vi "TDF - Time Varying Filter - Gabor.vi"(0 "reference in":refnum<class "GSwFormDSP.lvclass">, 5 "error in (no error)":errorcluster, 6 "Anotate Signal Name":bool=TRUE) -> (14 "reference in":refnum<class "GSwFormDSP.lvclass">, 19 "error out":errorcluster)   [LabVIEW 2022 SP3, in "GSwFormDSP.lvclass"]
uses:
  GSwFormDSP.lvclass
  <vilib>/addons/Time Frequency Analysis/Application.llb/TFA Time Varying Filter (Waveform).vi
  <vilib>/addons/_Advanced Signal Processing/NI_AdvSigProcTFA.lvlib
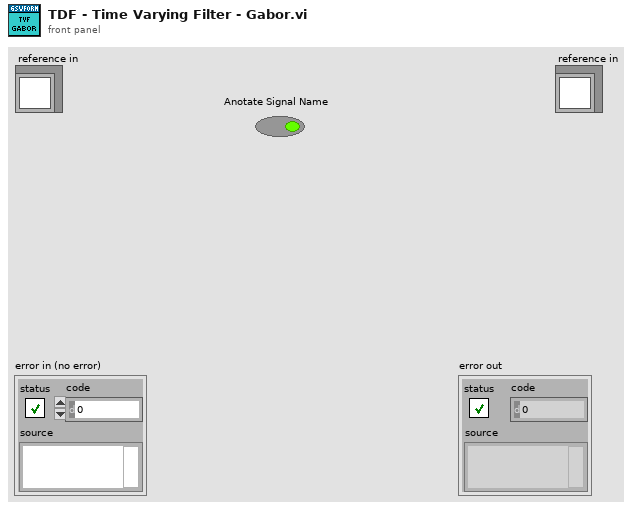
[diagram p1: front panel]
types:
  T1 = typedef "GSwFormDSP.lvclass/ObjectAttributes.ctl" = cluster{"Wform Ref":refnum<data-value>, "Nb Signals":i32, "Spectral Function Parameters":T2, "FFT":waveform(cdb)[], "Nb FFT":i32, "Nb Averages":i32[], "Reference Indexes":i32[], "Response Indexes":i32[], "Coherence":waveform(dbl)[], "TDF Parameters":T4, "DAQ":cluster{"Duration (sec)":dbl, "Buffer Size (Samples)":i32, "Offset (Samples)":i32}, "Filter Impulse Response (TDF)":waveform(dbl), "Sound Playback":T5}
  T2 = typedef "GSwFormDSP.lvclass/Spectral Parameters.ctl" = cluster{"Frequency resolution (Hz)":dbl, "Overlap":dbl, "Window":T3}
  T3 = typedef "NI_AALPro.lvlib/windowTd.ctl" = u32
  T4 = typedef "GSwFormDSP.lvclass/TDF Parameters.ctl" = cluster{"Filter":enum32{"Lowpass", "Highpass", "Bandpass", "Bandstop"}, "Type:":enum16{"Butterworth", "Chebyshev", "Inv Chebyshev", "Elliptic", "Bessel"}, "LP cutoff freq":dbl, "HP cutoff freq":dbl, "Order":i32, "passband ripple (dB)":dbl, "stopband attenuation (dB)":dbl, "Phaseless Filter":bool, "Include Fade IN and OUT":bool}
  T5 = typedef "GSwFormDSP.lvclass/Sound Playback.ctl" = cluster{"Timer start (ms)":u32, "task ID":T6, "Cursor Init Location (s)":dbl, "SC Volume":dbl}
  T6 = typedef "Sound Output Task ID.ctl" = u32
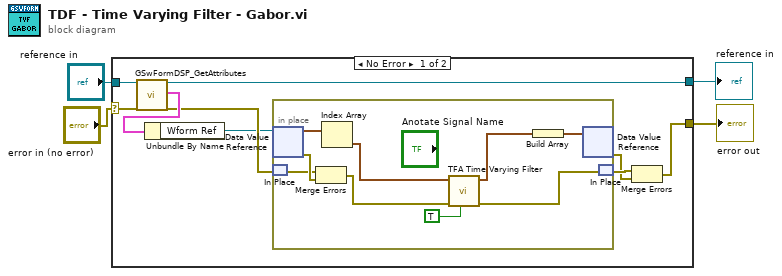
[diagram p0: block diagram]
diagram:
  n1 = case shown="No Error" "error in (no error)" {
    selector: "error in (no error)" -> [w11 w24]
    tunnel: [w13 w24] -> w3
    tunnel: [w9 w23] -> w2
    tunnel: "reference in" -> [w12 w23]
    frame No Error {
      n2 = call "GSwFormDSP_GetAttributes.vi"("reference in"=w12, "error in (no error)"=w11) -> ("reference out"=w9:refnum<class "GSwFormDSP.lvclass">, "attributes"=w10:T1, "error out"=w8:errorcluster)  [unwired: 14 in, 1 out]
      n3 = Unbundle By Name(w10) -> ("Wform Ref"=w7:refnum<data-value>)
      n4 = in-place {
        n5 = in-place-dvr #1(w7) -> (w20:waveform(dbl)[], w22:errorcluster)
        n6 = in-place-match #2(w8) -> (w21:errorcluster)
        n7 = Merge Errors(w21, w22) -> (w16:errorcluster)
        n8 = Index Array(array=w20) -> (element=w19:waveform(dbl))  [unwired: 1 in]
        n9 = call-poly <vilib>:"TFA Time Varying Filter.vi"("open front panel? (T)"=TRUE, "error in (no error)"=w16, "signal"=w19) -> ("error out"=w15:errorcluster, "filtered signal"=w17:waveform(dbl))  [unwired: 6 in, 1 out]
        n10 = Build Array(w17) -> (w18:waveform(dbl)[])
        n11 = in-place-dvr #1(w18) -> (w5:errorcluster)  [unwired: 1 out]
        n12 = in-place-match #2(w15) -> (w6:errorcluster)
      }
      n13 = Merge Errors(w6, w5) -> (w13:errorcluster)
    }
    frame Error {
    }
  }
  "error out" <- w3
  "reference in" <- w2
